vi "User Event List AE.vi"(7 "Action":enum16{"Set", "Get"}(ring), 11 "Event Structure Info (set)":T1[](array[typedef])) -> (3 "Event Structure Info Out":T1[](array[typedef]))   [LabVIEW 2021, in "TAF Proj Document Type.lvlib" / "Project Parser.lvlib"]
uses:
  <vilib>/Wovalab/AntiDoc/Document Type/Add-ons/LabVIEW TAF Project/Project Parser/Project Parser.lvlib
  <vilib>/Wovalab/AntiDoc/Document Type/Add-ons/LabVIEW TAF Project/Project Parser/User Event Info.ctl
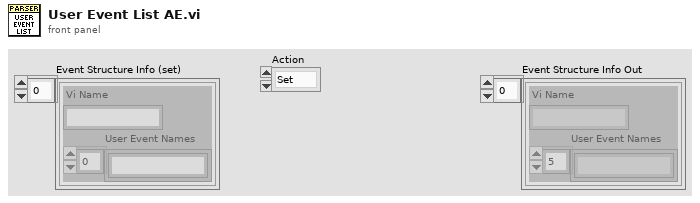
[diagram p1: front panel]
types:
  T1 = typedef "TAF Proj Document Type.lvlib/Project Parser.lvlib/User Event Info.ctl" = cluster{"Vi Name":string, "User Event Names":string[]}
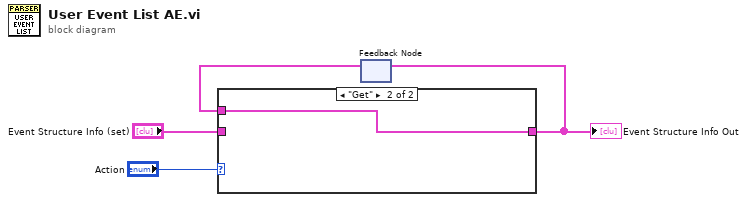
[diagram p0: block diagram]
diagram:
  n1 = feedback #1() -> (w1:T1[])  [unwired: 1 in]
  n2 = case shown="\"Get\"" "Action" {
    tunnel: [w5 w6] -> w2
    tunnel: "Event Structure Info (set)" -> [w5 _]
    tunnel: w1 -> [_ w6]
    frame "Set" {
    }
    frame "Get" {
    }
  }
  "Event Structure Info Out" <- w2
  n3 = feedback-in #1(w2) -> ()
